vi "UDP - Receiver.vi"() -> ()   [LabVIEW 2017]
doc: "The UDP protocol differs from TCP in that there is no error-checking with the packets of information that are sent, and thus no guarantee whatsoever that an intended recipient will actually receive a given piece of data.\n\nThis UDP Receiver VI connects to a port and reads and converts datagrams sent by VeriStand when running the system definition created by Import Data Sharing Framework with UDP Component VI."
panel:
  out "numerics (DBL)":dbl[](array[numeric]) format="%#_10f"
  out "unsigned byte array":u8[][](array[numeric])
  out "received string data":string
  in  "Stop":bool
  # "Overview: Demonstrates the use of the UDP functions to receive data over a UDP connection.\nInstructions:\n1. Run the Import Data Sharing Framework with UDP Component  example VI to configure VeriStand to send data to port 50001.\n2. Run this VI to read from receiver port 50001 using the UDP API and then convert data to the expected format."
  # "Van"
  # "Vbn"
  # "Vcn"
  # "Ia"
  # "Ib"
  # "Ic"
  # "In"
  # "Vdc"
  # "Idc"
  # "count"
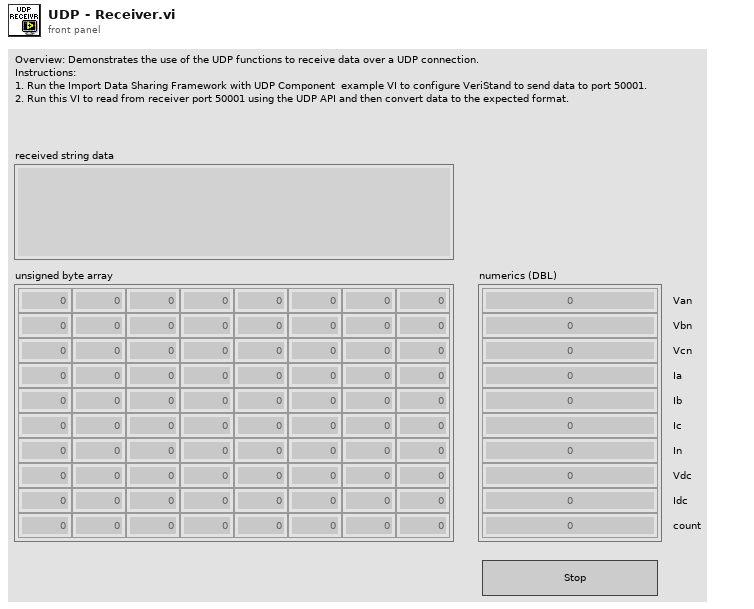
[diagram p1: front panel]
types:
  T1 = enum16{"big-endian, network order", "native, host order", "little-endian"}
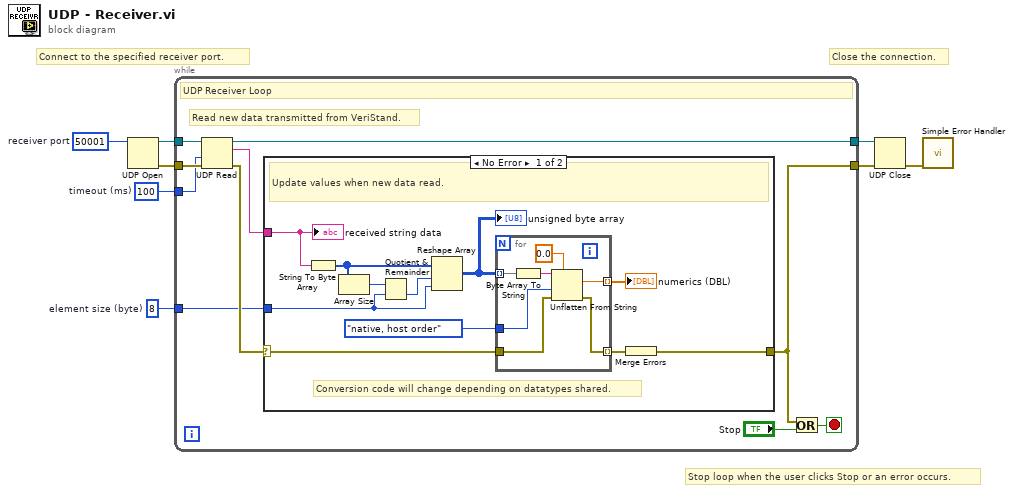
[diagram p0: block diagram]
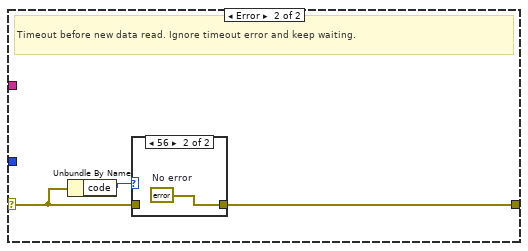
[diagram p2: hidden frame]
diagram:
  w1 = 8  # element size (byte)
  w2 = 100  # timeout (ms)
  w3 = u16 50001  # receiver port
  # "Stop loop when the user clicks Stop or an error occurs."
  # "Close the connection."
  # "Connect to the specified receiver port."
  n1 = UDP Open(11:w3) -> (port=w4:refnum<k16>, 0:w5:errorcluster)  [unwired: 4 in, 1 out]
  n2 = while {
    tunnel: w4 -> [w18]
    tunnel: [w11] -> w8
    tunnel: w5 -> [w15]
    tunnel: [w12] -> w6
    tunnel: w2 -> [w10]
    tunnel: w1 -> [w9]
    stop <- w16 stop-if-true
    # "Read new data transmitted from VeriStand."
    # "UDP Receiver Loop"
    n3 = UDP Read(connection ID=w18, timeout ms (25000)=w10, 8:w15) -> (data out=w14:string, error out=w13:errorcluster, 3:w11:refnum<k16>)  [unwired: 3 out]
    n4 = case shown="No Error" w13 {
      selector: w13 -> [w19 w38]
      tunnel: w14 -> [w29 _]
      tunnel: [w23 w37] -> w12
      tunnel: w9 -> [w25 _]
      frame No Error {
        # "Conversion code will change depending on datatypes shared."
        # "Update values when new data read."
        n5 = String To Byte Array(string=w29) -> (unsigned byte array=w27:u8[])
        n6 = Array Size(array=w27) -> (size(s)=w28:i32)
        n7 = Quotient & Remainder(x=w28, y=w25) -> (floor(x/y)=w26:i32)  [unwired: 1 out]
        n8 = Reshape Array(w27, w26, w25) -> (w22:u8[][])
        "unsigned byte array" <- w22
        n9 = for {
          tunnel: w22 -> [w36] mode=indexing
          tunnel: [w34] -> w21 mode=indexing
          tunnel: w19 -> [w32]
          tunnel: [w31] -> w24 mode=indexing
          tunnel: T1."native, host order" ("byte order (0:big-endian, network order)") -> [w30]
          n10 = Byte Array To String(unsigned byte array=w36) -> (string=w35:string)
          n11 = Unflatten From String(type=0.0, binary string=w35, byte order (0:big-endian, network order)=w30, error in (no error)=w32) -> (value=w34:dbl, error out=w31:errorcluster)  [unwired: 1 in, 1 out]
        }
        "numerics (DBL)" <- w21
        n12 = Merge Errors(w24) -> (w23:errorcluster)
        "received string data" <- w29
      }
      frame Error {
        # "Timeout before new data read. Ignore timeout error and keep waiting."
        n13 = Unbundle By Name(w38) -> ("code"=w39:i32)
        n14 = case shown="56" w39 {
          tunnel: w38 -> [w40 _]
          tunnel: [w40 w41] -> w37
          frame Default {
          }
          frame 56 {
            w41 = errorcluster {"status"=FALSE, "code"=0, "source"=""}  # No error
          }
        }
      }
    }
    n15 = Or(x=w12, y="Stop") -> (x .or. y?=w16:bool)
  }
  n16 = UDP Close(connection ID=w8, 8:w6) -> (error out=w7:errorcluster)  [unwired: 1 out]
  n17 = call <vilib>:"Simple Error Handler.vi"("error in (no error)"=w7) -> ()  [unwired: 1 in, 8 out]
